vi "Initialise parameters.vi"(8 "error in (no error)":errorcluster, 11 "DAQMH121119OrcaFlash in":refnum<class "DAQOrcaFlash.lvclass">) -> (0 "error out":errorcluster, 3 "DAQMH121119OrcaFlash out":refnum<class "DAQOrcaFlash.lvclass">)   [LabVIEW 2012, in "DAQOrcaFlash.lvclass"]
uses:
  DAQOrcaFlash.lvclass
  DAQOrcaFlash.lvclass/DAQOrcaFlash.ctl
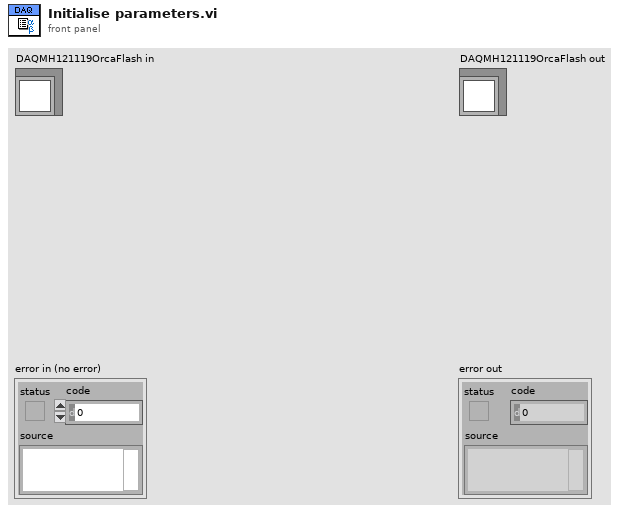
[diagram p1: front panel]
types:
  T1 = enum8{"Enabled", "Disabled", "Disabled and Grayed Out"}
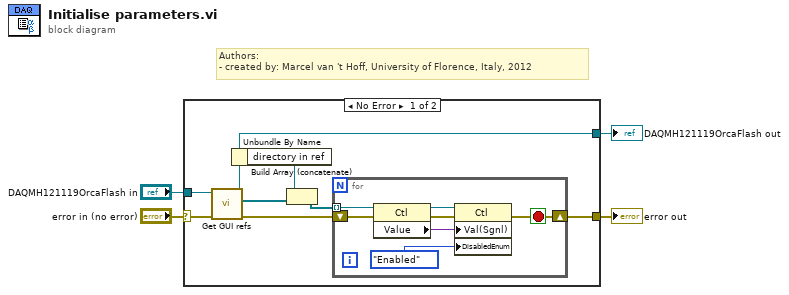
[diagram p0: block diagram]
diagram:
  # "Authors: \n- created by: Marcel van 't Hoff, University of Florence, Italy, 2012"
  n1 = case shown="No Error" "error in (no error)" {
    selector: "error in (no error)" -> [w8 w21]
    tunnel: [w11 w21] -> w3
    tunnel: [w5 w20] -> w1
    tunnel: "DAQMH121119OrcaFlash in" -> [w9 w20]
    frame No Error {
      n2 = call "Get GUI refs.vi"("error in (no error)"=w8, "DAQMH121119OrcaFlash in"=w9) -> ("error out"=w7:errorcluster, "Array"=w10:refnum<vi>[], "DAQMH121119OrcaFlash out"=w5:refnum<class "DAQOrcaFlash.lvclass">)  [unwired: 7 in]
      n3 = Unbundle By Name(w5) -> ("directory in ref"=w6:refnum<vi>)
      n4 = Build Array (concatenate)(w6, w10) -> (w12:refnum<vi>[])
      n5 = for {
        tunnel: w12 -> [w19] mode=indexing
        shift-right: [w15] -> w11
        shift-left: w7 -> [w16]
        stop <- w15 stop-if-true
        n6 = property class="Ctl"(reference=w19, error in=w16) -> (reference out=w18:refnum<vi>, error out=w14:errorcluster, "Value"=w17:variant)
        n7 = property class="Ctl"(reference=w18, error in=w14, "Val(Sgnl)"=w17, "DisabledEnum"=T1."Enabled" ("Disabled")) -> (error out=w15:errorcluster)  [unwired: 1 out]
      }
    }
    frame Error {
    }
  }
  "error out" <- w3
  "DAQMH121119OrcaFlash out" <- w1
